vi "Setup Data Acquisition.vi"(4 "error in (no error)":errorcluster, 6 "Data Acquisition Parameters":T1={"Data acquisition mode"=0, "Axis used to trigger data acquisition (1)"=1, "Data acquisition parameter 3 (=0)"=0, "Position feedback channels"=0, "Data acquisition rate (0=400µs)"=0, "Number of data sample to be acquired (0)"=1} {"Number of data sample to be acquired (0)" min=1 max=1000 format="%#.0f"; "Data acquisition rate (0=400µs)" max=1000 format="%#.0f"; "Position feedback channels" items=["None", "channel 1", "channel 2", "channel 1 & 2", "channel 3", "channel 1 & 3", "channel 2 & 4", "channel 1, 2 & 3"]; "Data acquisition parameter 3 (=0)" max=0 format="%#.0f"; "Axis used to trigger data acquisition (1)" min=1 max=3 format="%#.0f"; "Data acquisition mode" items=["Start immediately", "Start when trigger axis starts motion", "Start when trigger axis reaches slew speed"]}, 7 "VISA resource name":refnum<visa-resource-name>) -> (0 "error out":errorcluster, 3 "VISA resource name out":refnum<visa-resource-name>)   [LabVIEW 2010, in "Newport ESP301.lvlib"]
doc: "This command is used to setup data acquisition—analog data acquisition (ADC) as well as acquisition of certain trace variables—using ESP motion controller.\n<B> Data Acquisition Mode (0)</B>: Data acquisition modes 0—2 support different ways in which analog data can be collected. \n 0: Start data acquisition immediately\n 1: Start data acquisition when trigger axis starts motion\n 2: Start data acquisition when trigger axis reaches slew speed\n<B> Axis used to trigger data acquisition (1) </B>:: Data acquisition is triggered by the motion of an axis specified through this parameter. Exceptions to this requirement are in the case of data acquisition mode 0. For thiscases enabling data acquisition is sufficient to start the data acquisition process. For all other modes, two conditions—enabling of data acquisition and any mode dependent conditions such as trigger axis starting motion or reaching slew speed—must be met in order to start the data acquisition process.\n<B> Data acquisition parameter 3 (=0) </B>: set this value to 0.\n<B> Position feedback channels collected(0) </B>: Identifies the position feedback channels to be collected.\n 0 : None\n 1 : channel 1\n 2 : channel 2\n 3 : channel 1 & 2\n 4 : channel 3\n 5 : channel 1 & 3\n 6 : channel 2 & 4\n 7 : channel 1, 2 & 3\n<B> Data acquisition rate(0=400µs) </B>: The rate at which data is to be acquired is specified through this parameter. The rate specified is in multiples of the (400 µs) rate. For example, a value of 0 implies data acquisition every servo cycle (400 µs), a value of 1 implies every other servo cycle (400 µs), and so on.\n<B> Number of data sample to be acquired(0) </B>: The number of samples of data to be acquired is specified through this parameter. Data acquisition process is considered to be \"done\" only after the number of samples specified by this parameter are acquired by the controller. The status of data acquisition process may be found by issuing ASCII command, DD. Once the data acquisition is done, ASCII command, DG may be used to collect the data from the controller.\n\n<B>Note</B>: The controller responds with a servo cycle (400 µs) tick count along with every data sample collected."
uses:
  <userlib>/Newport ESP301/Newport ESP301.lvlib
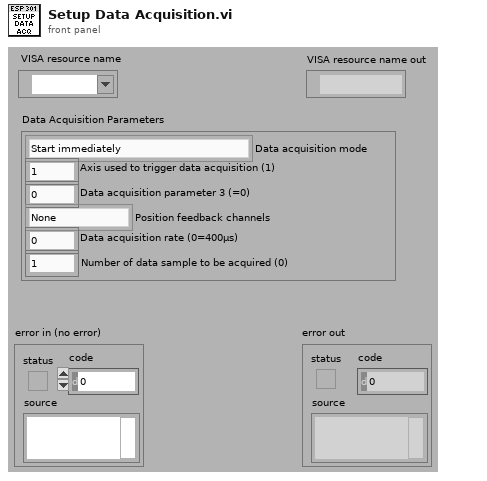
[diagram p1: front panel]
types:
  T1 = cluster{"Data acquisition mode":u32, "Axis used to trigger data acquisition (1)":u32, "Data acquisition parameter 3 (=0)":u32, "Position feedback channels":u32, "Data acquisition rate (0=400µs)":u32, "Number of data sample to be acquired (0)":u32}
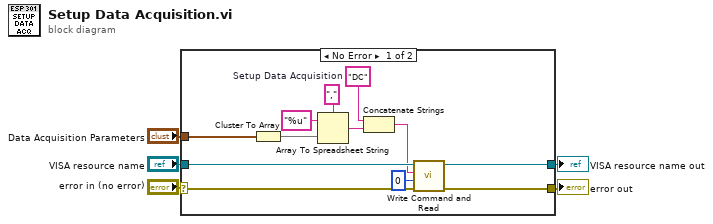
[diagram p0: block diagram]
diagram:
  n1 = case shown="No Error" "error in (no error)" {
    selector: "error in (no error)" -> [w16 w19]
    tunnel: [w13 w19] -> w4
    tunnel: "VISA resource name" -> [w17 w18]
    tunnel: [w14 w18] -> w2
    tunnel: "Data Acquisition Parameters" -> [w7 _]
    frame No Error {
      w10 = "DC"  # Setup Data Acquisition
      n2 = Cluster To Array(cluster=w7) -> (array=w6:u32[])
      n3 = Array To Spreadsheet String(delimiter (Tab)="," ("séparateur (Tabulation)"), array=w6, 3:"%u" ("chaîne de format")) -> (spreadsheet string=w11:string)
      n4 = Concatenate Strings(w10, w11) -> (w8:string)
      n5 = call <userlib>:"Write Command and Read.vi"("error in (no error)"=w16, "Bytes to read (100)"=u32 0, "Command"=w8, "VISA resource name"=w17) -> ("error out"=w13:errorcluster, "VISA resource name out"=w14:refnum<visa-resource-name>)  [unwired: 1 in, 3 out]
    }
    frame Error {
    }
  }
  "error out" <- w4
  "VISA resource name out" <- w2
